vi "Build COM Table INI.vi"() -> ()   [LabVIEW 2015, in "RDS Configuration Library.lvlib"]
uses:
  Configuration Library/RDS Configuration Library.lvlib
  RDS Instruments/COM Port Table.ctl
panel:
  in  "Close":bool
  out "COM Port Table":T1
  in  "Read":bool
  in  "COM Port Table":T1
  in  "Write":bool
  out "Array":string[](array[string])
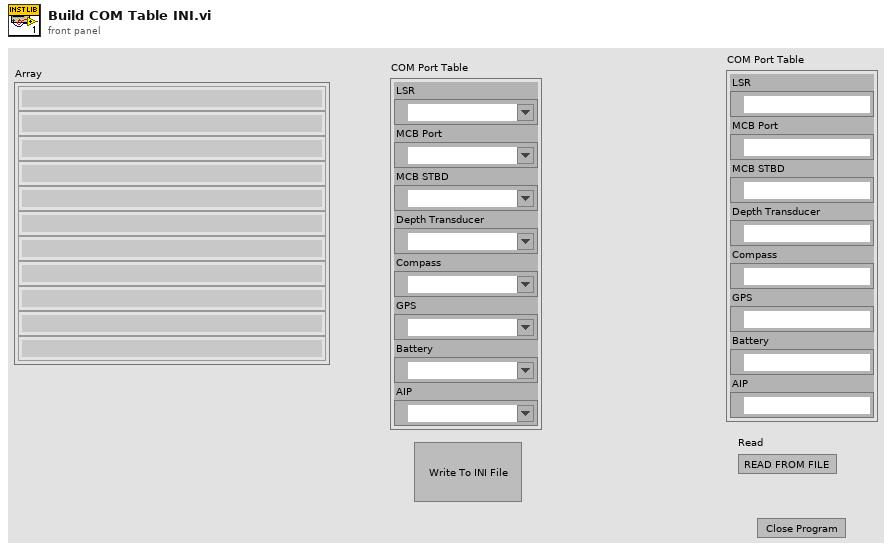
[diagram p1: front panel]
types:
  T1 = typedef "RDS Configuration Library.lvlib/COM Port Table.ctl" = cluster{"LSR":refnum<visa-resource-name>, "MCB Port":refnum<visa-resource-name>, "MCB STBD":refnum<visa-resource-name>, "Depth Transducer":refnum<visa-resource-name>, "Compass":refnum<visa-resource-name>, "GPS":refnum<visa-resource-name>, "Battery":refnum<visa-resource-name>, "AIP":refnum<visa-resource-name>}
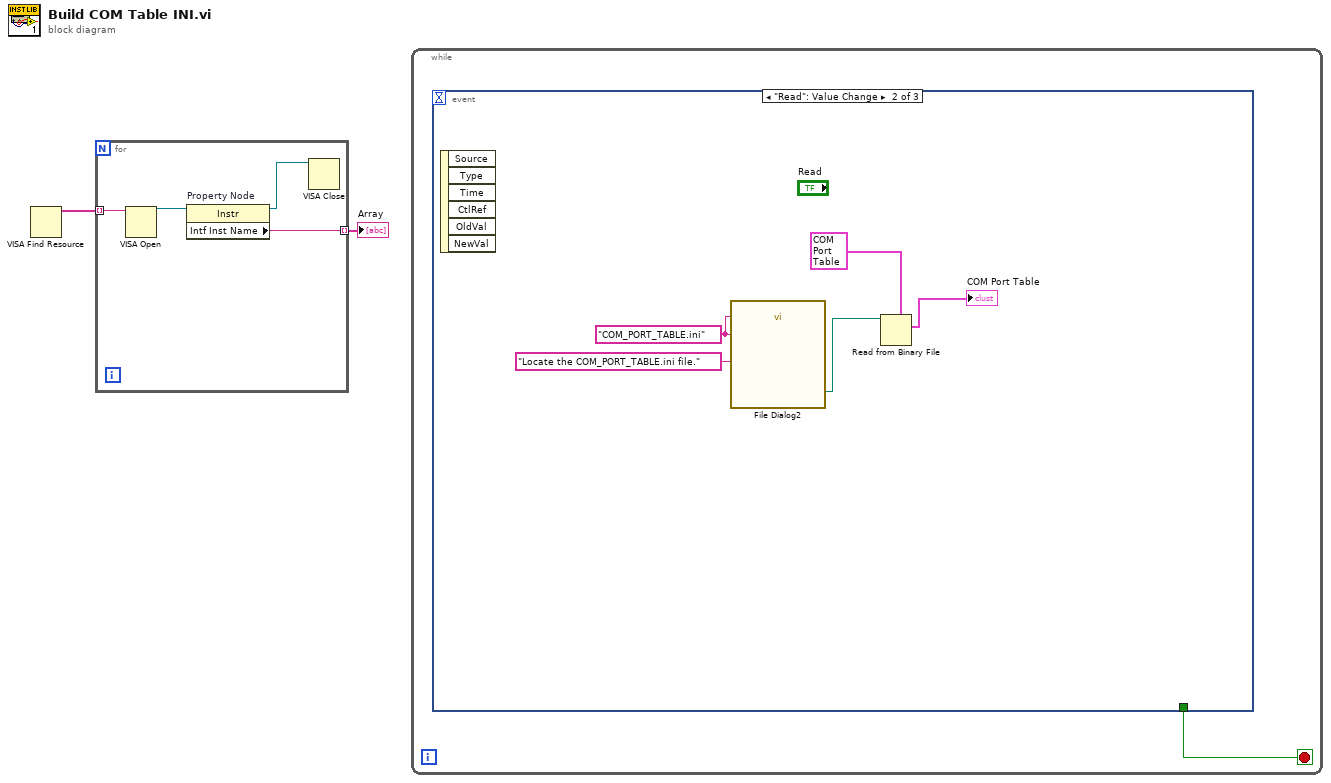
[diagram p0: block diagram]
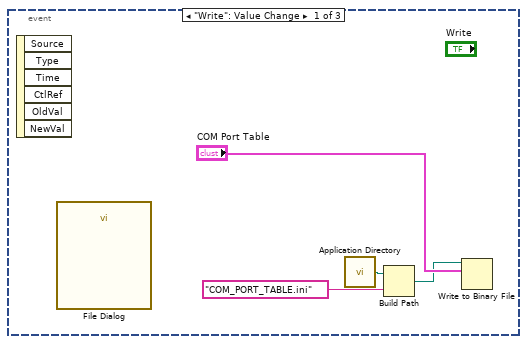
[diagram p2: hidden frame]
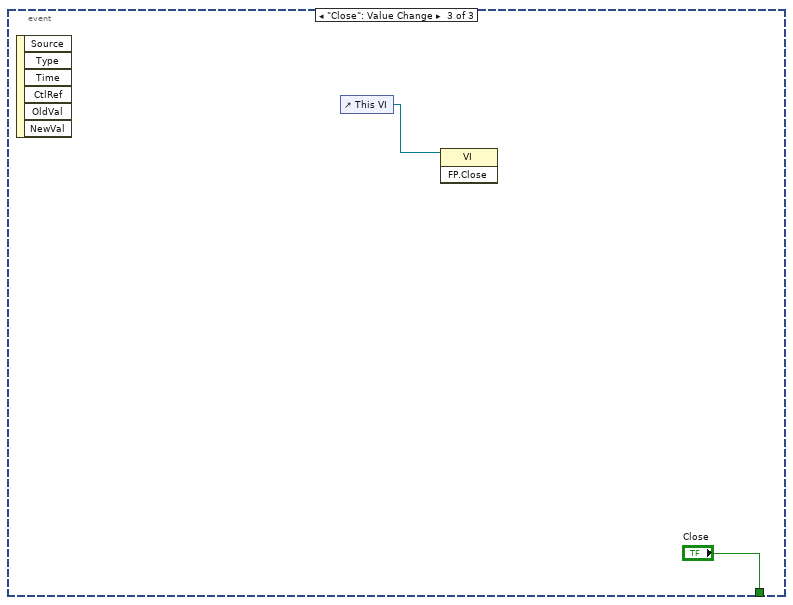
[diagram p3: hidden frame]
diagram:
  n1 = VISA Find Resource() -> (3:w2:string[])  [unwired: 3 in, 2 out]
  n2 = for {
    tunnel: w2 -> [w6] mode=indexing
    tunnel: [w4] -> w1 mode=indexing
    n3 = VISA Open(VISA resource name=w6) -> (VISA resource name=w5:refnum<visa-resource-name>)  [unwired: 4 in, 1 out]
    n4 = property on="Property Node" class="Instr"(reference=w5) -> (reference out=w3:refnum<visa-resource-name>, "Intf Inst Name"=w4:string)  [unwired: 1 in, 1 out]
    n5 = VISA Close(VISA resource name=w3) -> ()  [unwired: 1 in, 1 out]
  }
  "Array" <- w1
  n6 = while {
    stop <- w7 stop-if-true
    n7 = event shown="[1] \"Read\": Value Change" {
      selector: _ -> [_ _ _]
      dyn-events: _ -> [_ _ _]
      timeout: _ -> [_ _ _]
      tunnel: [_ _ "Close"] -> w7
      event "Write": Value Change {
        n8 = event-data() -> ()  [unwired: 1 in, 6 out]
        n9 = call "File Dialog"() -> ()  [unwired: 12 in, 4 out]
        n10 = call <vilib>:"Application Directory.vi"() -> ("Application Directory"=w10:path)
        n11 = Build Path(base path=w10, name or relative path="COM_PORT_TABLE.ini") -> (appended path=w8:path)
        n12 = Write to Binary File(file (use dialog)=w8, data="COM Port Table") -> ()  [unwired: 4 in, 3 out]
      }
      event "Read": Value Change {
        w13 = "COM_PORT_TABLE.ini" ("pattern (all files)")
        n13 = event-data() -> ()  [unwired: 1 in, 6 out]
        n14 = call "File Dialog2"("prompt"="Locate the COM_PORT_TABLE.ini file.", "default name"=w13, "pattern (all files)"=w13) -> ("selected path"=w14:path)  [unwired: 9 in, 3 out]
        n15 = Read from Binary File(5:T1 {"LSR"="COM1", "MCB Port"="COM2", "MCB STBD"="COM3", "Depth Transducer"="COM4", "Compass"="COM5", "GPS"="COM6", "Battery"="COM7", "AIP"="COM10"} ("COM Port Table"), 11:w14) -> (2:→"COM Port Table":T1)  [unwired: 4 in, 3 out]
      }
      event "Close": Value Change {
        n16 = event-data() -> ()  [unwired: 1 in, 6 out]
        n17 = control-ref of="This VI"() -> (w18:refnum<vi>)
        n18 = invoke class="VI" method="FP.Close"(reference=w18) -> ()  [unwired: 2 in, 3 out]
      }
    }
  }
